vi "SpeedAccelDistanceM1M2_2.vi"(0 "VISA Refnum in":refnum<visa-resource-name>, 1 "Accel1":u32 max=127 step=1, 2 "Speed1":i32 max=127 step=1, 3 "Distance1":u32 max=127 step=1, 5 "Address":u8, 8 "Accel2":u32 max=127 step=1, 10 "Speed2":i32 max=127 step=1, 11 "error in (no error)":errorcluster, 14 "Distance2":u32 max=127 step=1) -> (4 "VISA Refnum out":refnum<visa-resource-name>, 6 "Valid":bool, 15 "error out":errorcluster)   [LabVIEW 2015, in "Ion Motion Roboclaw.lvlib"]
uses:
  <instrlib>/Ion Motion Roboclaw/Ion Motion Roboclaw.lvlib
panel:
  in  "Immediate":u8 max=127 step=1
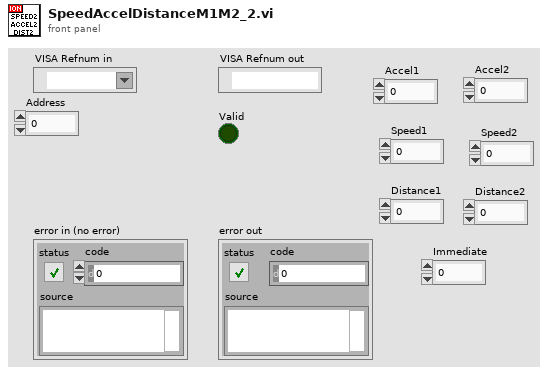
[diagram p1: front panel]
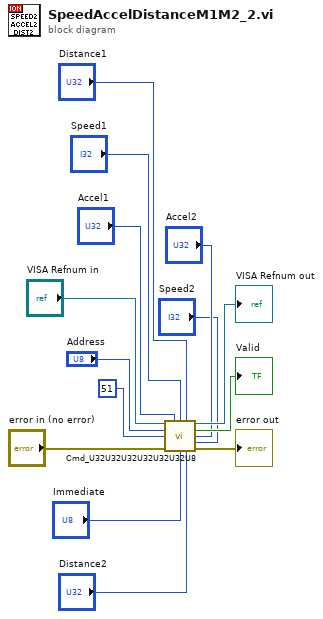
[diagram p0: block diagram]
diagram:
  n1 = call <instrlib>:"Cmd_U32U32U32U32U32U32U8.vi"("VISA Refnum in"="VISA Refnum in", "Arg1"="Accel1", "Arg2"="Speed1", "Arg3"="Distance1", "Address"="Address", "Cmd"=u8 51, "Arg4"="Accel2", "Arg5"="Speed2", "error in (no error)"="error in (no error)", "Arg7"="Immediate", "Arg6"="Distance2") -> ("VISA Refnum out"=→"VISA Refnum out":refnum<visa-resource-name>, "Valid"=→"Valid":bool, "error out"=→"error out":errorcluster)  [unwired: 2 in]
